vi "Observer_Create.vi"(0 "reference in":refnum<class "Observer.lvclass">, 5 "error in (no error)":errorcluster) -> (14 "reference out":refnum<class "Observer.lvclass">, 19 "error out":errorcluster)   [LabVIEW 2010, in "Observer.lvclass"]
uses:
  Observer.lvclass
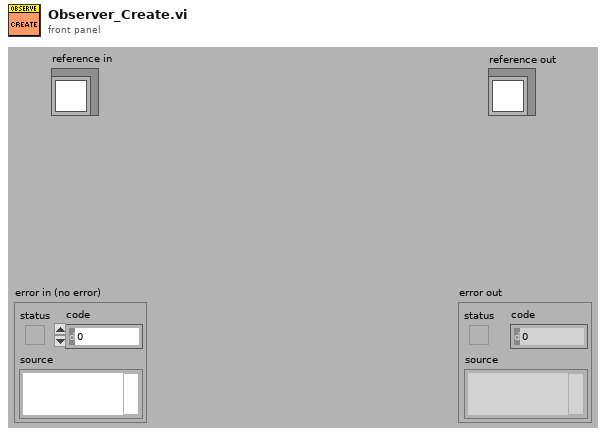
[diagram p1: front panel]
types:
  T1 = typedef "G4BaseTemplate_Simple_6x8x6.lvclass/ObjectAttributes.ctl" = cluster{"Attribute1":dbl}
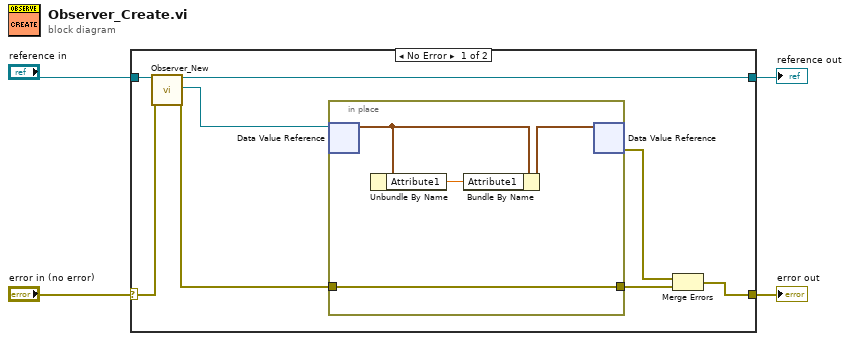
[diagram p0: block diagram]
diagram:
  n1 = case shown="No Error" "error in (no error)" {
    selector: "error in (no error)" -> [w11 w18]
    tunnel: [w8 w18] -> w3
    tunnel: "reference in" -> [w12 w17]
    tunnel: [w10 w17] -> w1
    frame No Error {
      n2 = call "Observer_New.vi"("reference in"=w12, "error in (no error)"=w11) -> ("reference out"=w10:refnum<class "Observer.lvclass">, "DVRRefOut"=w7:refnum<data-value>, "error out"=w6:errorcluster)  [unwired: 14 in, 1 out]
      n3 = in-place {
        in-place-border: w6 -> [w13]
        in-place-border: [w13] -> w5
        n4 = in-place-dvr #1(w7) -> (w15:T1)  [unwired: 1 out]
        n5 = Unbundle By Name(w15) -> ("Attribute1"=w14:dbl)
        n6 = Bundle By Name(cluster=w15, "Attribute1"=w14) -> (w16:T1)
        n7 = in-place-dvr #1(w16) -> (w9:errorcluster)  [unwired: 1 out]
      }
      n8 = Merge Errors(w9, w5) -> (w8:errorcluster)
    }
    frame Error {
    }
  }
  "error out" <- w3
  "reference out" <- w1
